vi "find_objects.vi"(6 "objects finding parameters in":T1={"Objects"=0, "Threshold"=6700, "Reject Border"=TRUE, "Fill Holes"=FALSE, "Min Object Size"=FALSE, "Min Size"=30, "Max Object Size"=FALSE, "Max Size"=100, "Show Search Area"=FALSE, "Show Center"=FALSE, "Show Bounding Box"=TRUE} {"Objects" items=["Bright Objects", "Dark Objects"]}, 7 "expected size in pixels":dbl=3.0, 8 "error in":errorcluster, 10 "array in":u16[][](array[numeric])) -> (0 "error out":errorcluster, 2 "regions found with fit parameters":T2[](array[typedef]))   [LabVIEW 2010]
uses:
  object_parameters.ctl
panel:
  out "Image 2":T3(plugin-control)
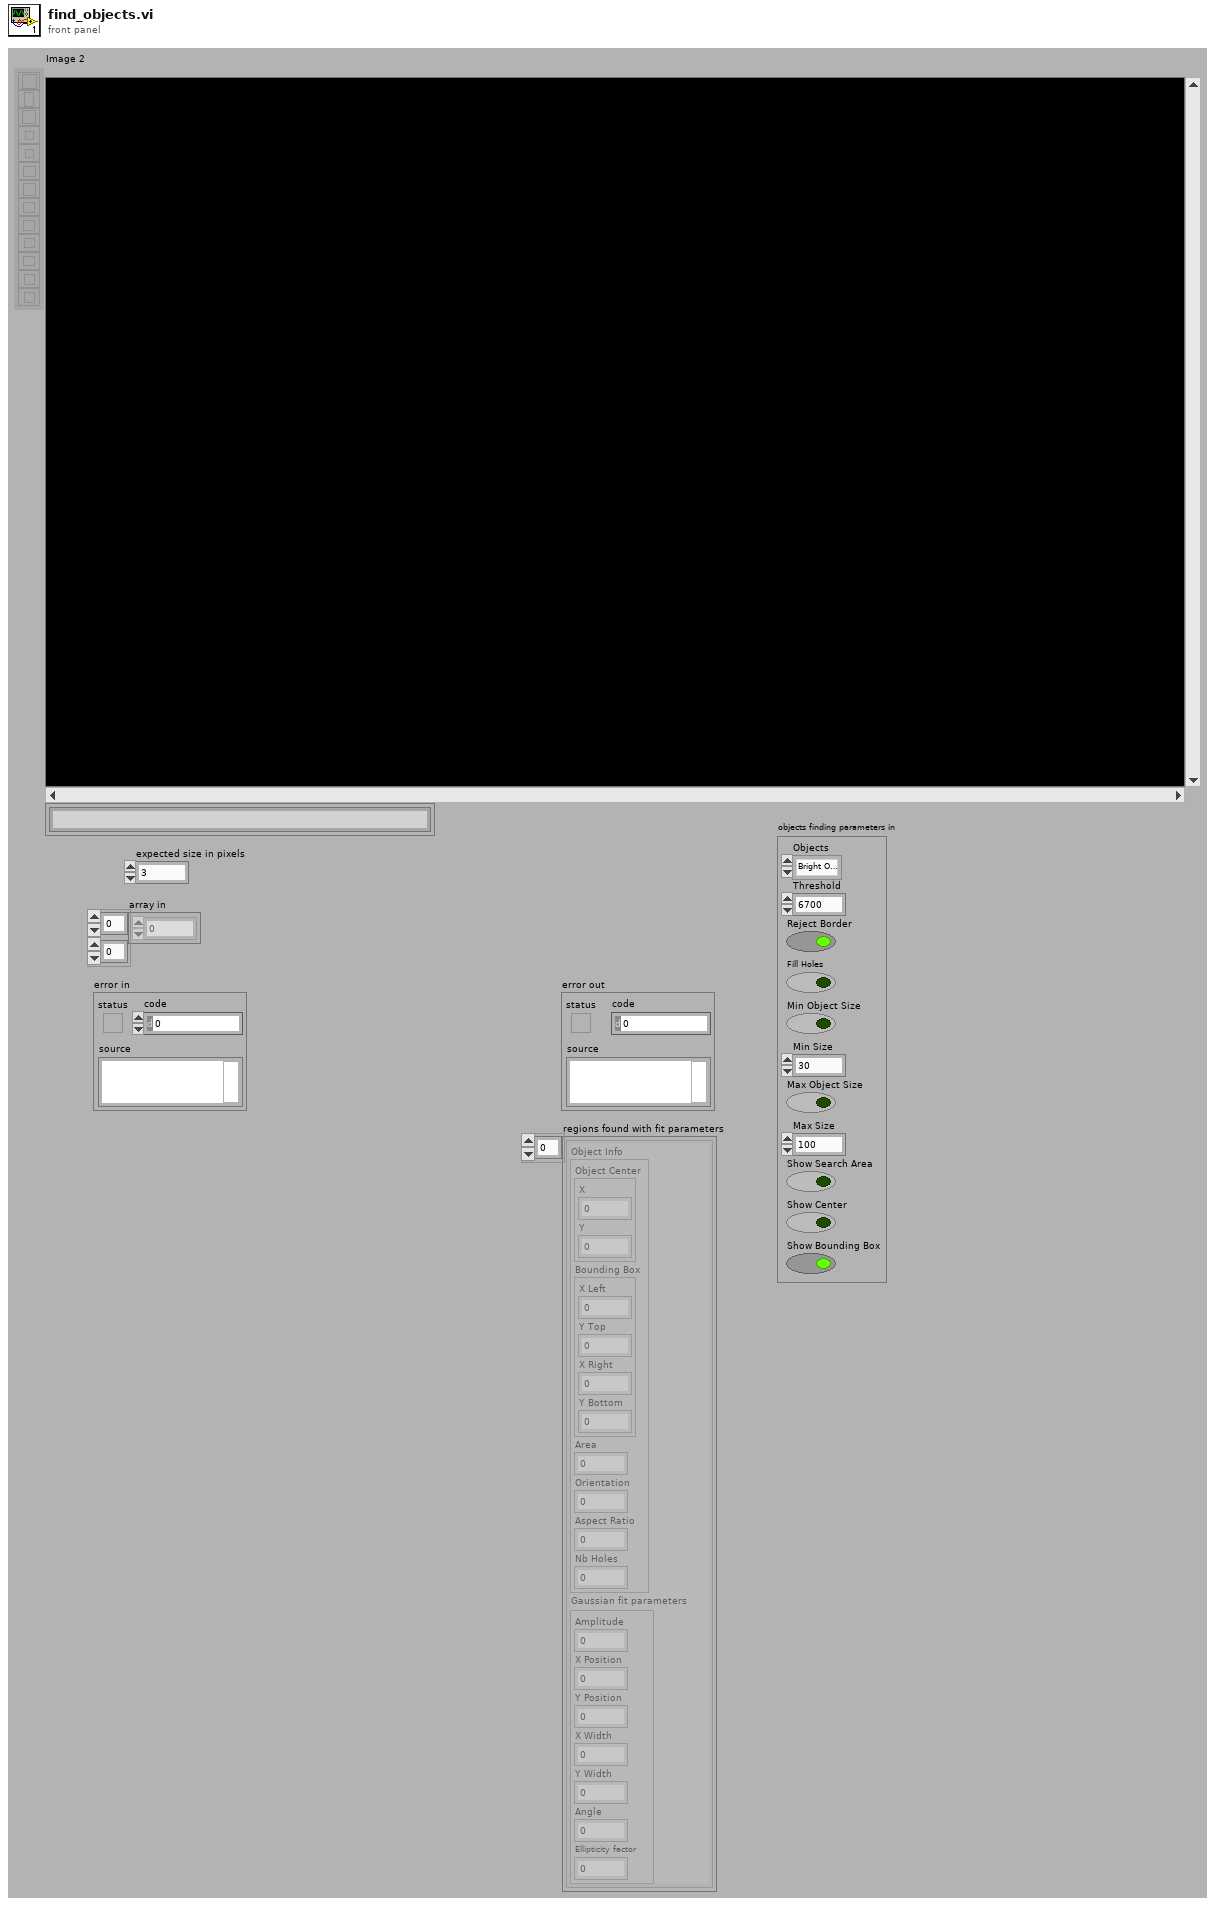
[diagram p1: front panel]
types:
  T1 = cluster{"Objects":u16, "Threshold":i32, "Reject Border":bool, "Fill Holes":bool, "Min Object Size":bool, "Min Size":i32, "Max Object Size":bool, "Max Size":i32, "Show Search Area":bool, "Show Center":bool, "Show Bounding Box":bool}
  T2 = typedef "object_parameters.ctl" = cluster{"Object Info":cluster{"Object Center":cluster{"X":sgl, "Y":sgl}, "Bounding Box":cluster{"X Left":i32, "Y Top":i32, "X Right":i32, "Y Bottom":i32}, "Area":sgl, "Orientation":sgl, "Aspect Ratio":sgl, "Nb Holes":i32}, "Gaussian fit parameters":cluster{"Amplitude":dbl, "X Position":dbl, "Y Position":dbl, "X Width":dbl, "Y Width":dbl, "Angle":dbl, "Ellipticity factor":dbl}}
  T3 = typedef "IMAQ Image.ctl" = refnum<image>
  T4 = typedef "Image Type" = u32
  T5 = cluster{"Object Center":cluster{"X":sgl, "Y":sgl}, "Bounding Box":cluster{"X Left":i32, "Y Top":i32, "X Right":i32, "Y Bottom":i32}, "Area":sgl, "Orientation":sgl, "Aspect Ratio":sgl, "Nb Holes":i32}[]
  T6 = cluster{"best fit parameters[0]":dbl, "best fit parameters[1]":dbl, "best fit parameters[2]":dbl, "best fit parameters[3]":dbl, "best fit parameters[4]":dbl, "best fit parameters[5]":dbl, "best fit parameters[6]":dbl}
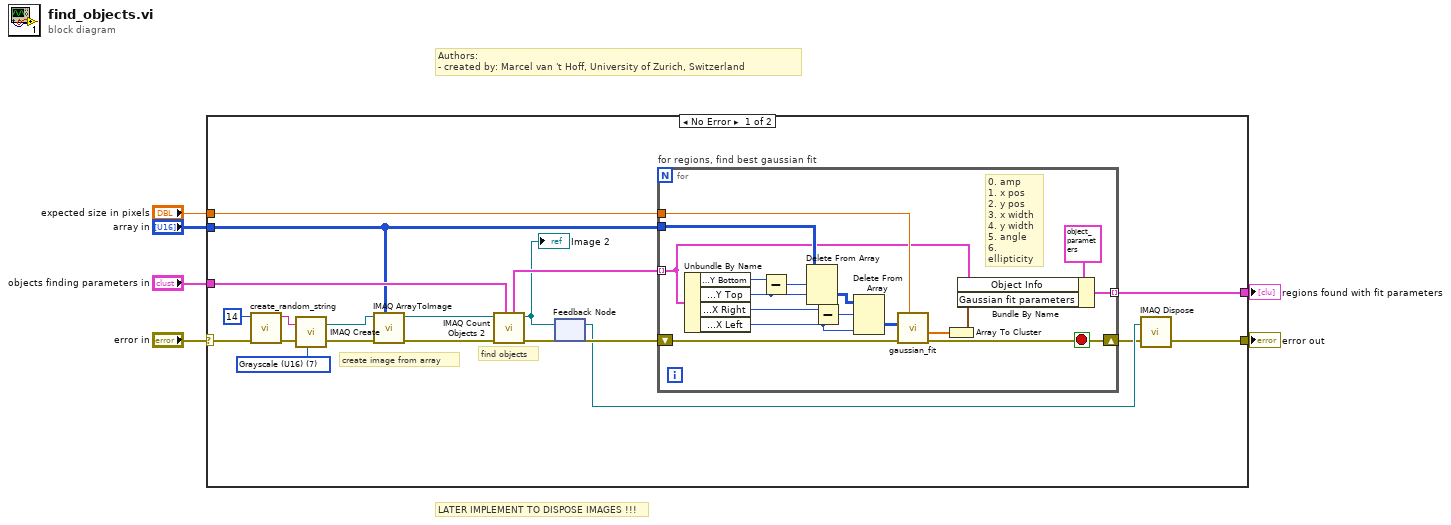
[diagram p0: block diagram]
diagram:
  # "LATER IMPLEMENT TO DISPOSE IMAGES !!!"
  # "Authors: \n- created by: Marcel van 't Hoff, University of Zurich, Switzerland"
  n1 = case shown="No Error" "error in" {
    selector: "error in" -> [w13 w43]
    tunnel: [w7 w43] -> w6
    tunnel: "array in" -> [w15 _]
    tunnel: "expected size in pixels" -> [w19 _]
    tunnel: [w18 _] -> w2
    tunnel: "objects finding parameters in" -> [w16 _]
    frame No Error {
      w20 = T4 7 items=["Grayscale (U8)", "Grayscale (I16)", "Grayscale (SGL)", "Complex (CSG)", "RGB (U32)", "HSL (U32)", "RGB (U64)", "Grayscale (U16)"] ("Image Type")
      # "create image from array"
      # "find objects"
      n2 = call "create_random_string.vi"("error in (no error)"=w13, "length"=14) -> ("error out"=w12:errorcluster, "random string"=w14:string)  [unwired: 8 in]
      n3 = call "IMAQ Create"("Image Name"=w14, "Image Type"=w20, "error in (no error)"=w12) -> ("New Image"=w21:T3, "error out"=w25:errorcluster)  [unwired: 2 in]
      n4 = call "IMAQ ArrayToImage"("Image Pixels (U16)"=w15, "error in (no error)"=w25, "Image"=w21) -> ("error out"=w24:errorcluster, "Image Out"=w22:T3)  [unwired: 7 in]
      n5 = call "IMAQ Count Objects 2"("Settings"=w16, "error in (no error)"=w24, "Image"=w22) -> ("error out"=w10:errorcluster, "Image Out"=w17:T3, "Objects"=w23:T5)  [unwired: 4 in, 2 out]
      "Image 2" <- w17
      n6 = feedback-in #1(w17) -> ()
      n7 = feedback #1() -> (w9:T3)  [unwired: 1 in]
      n8 = for "for regions, find best gaussian fit" {
        tunnel: w15 -> [w42]
        tunnel: w23 -> [w29] mode=indexing
        tunnel: w19 -> [w41]
        shift-right: [w31] -> w8
        shift-left: w10 -> [w32]
        tunnel: [w27] -> w18 mode=indexing
        stop <- w31 stop-if-true
        # "0. amp\n1. x pos\n2. y pos\n3. x width\n4. y width\n5. angle\n6. ellipticity"
        n9 = Unbundle By Name(w29) -> ("Bounding Box.Y Bottom"=w38:i32, "Bounding Box.Y Top"=w40:i32, "Bounding Box.X Right"=w36:i32, "Bounding Box.X Left"=w35:i32)
        n10 = Subtract(x=w38, y=w40) -> (x-y=w39:i32)
        n11 = Delete From Array(array=w42, length=w39, index (row)=w40) -> (deleted portion=w37:u16[][])  [unwired: 1 in, 1 out]
        n12 = Subtract(x=w36, y=w35) -> (x-y=w34:i32)
        n13 = Delete From Array(array=w37, length=w34, index (col)=w35) -> (deleted portion=w33:u16[][])  [unwired: 1 in, 1 out]
        n14 = call "gaussian_fit.vi"("expected size in pixels"=w41, "error in (no error)"=w32, "all rows"=w33) -> ("error out"=w31:errorcluster, "best fit parameters"=w28:dbl[])  [unwired: 6 in, 1 out]
        n15 = Array To Cluster(array=w28) -> (cluster=w26:T6)
        n16 = Bundle By Name(cluster=T2 {"Object Info"={"Object Center"={"X"=0.0, "Y"=0.0}, "Bounding Box"={"X Left"=0, "Y Top"=0, "X Right"=0, "Y Bottom"=0}, "Area"=0.0, "Orientation"=0.0, "Aspect Ratio"=0.0, "Nb Holes"=0}, "Gaussian fit parameters"={"Amplitude"=0.0, "X Position"=0.0, "Y Position"=0.0, "X Width"=0.0, "Y Width"=0.0, "Angle"=0.0, "Ellipticity factor"=0.0}} ("Object Info"), "Object Info"=w29, "Gaussian fit parameters"=w26) -> (w27:T2)
      }
      n17 = call "IMAQ Dispose"("Image"=w9, "error in (no error)"=w8) -> ("error out"=w7:errorcluster)  [unwired: 4 in]
    }
    frame Error {
    }
  }
  "error out" <- w6
  "regions found with fit parameters" <- w2
